vi "Desplegar arreglos boleanos.vi"(8 "error in (no error)":errorcluster, 10 "Expected Response out":string, 11 "Simulado in":refnum<class "Simulado.lvclass">) -> (0 "error out":errorcluster, 1 "Puerto":string, 2 "output array":bool[](array[boolean]), 3 "Simulado out":refnum<class "Simulado.lvclass">)   [LabVIEW 2020, in "Simulado.lvclass"]
uses:
  Simulado.lvclass
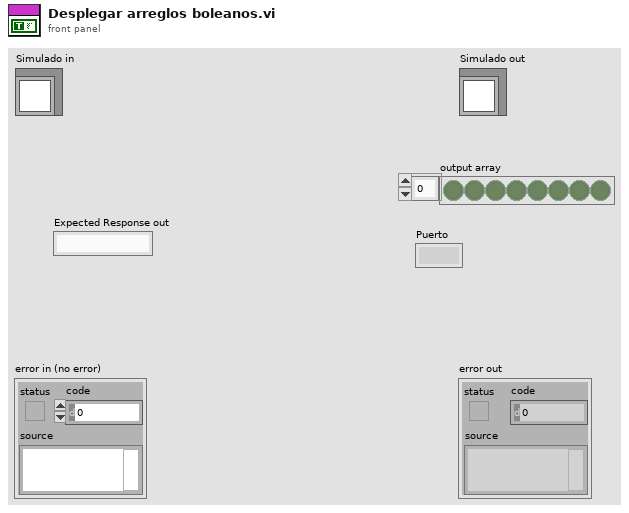
[diagram p1: front panel]
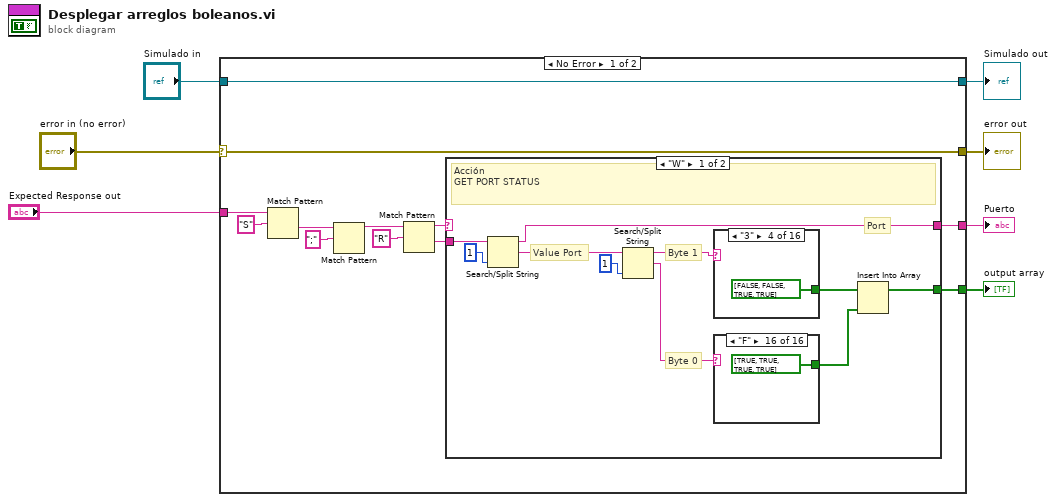
[diagram p0: block diagram]
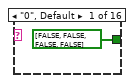
[diagram p2: hidden frame]
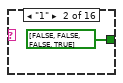
[diagram p3: hidden frame]
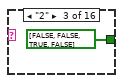
[diagram p4: hidden frame]
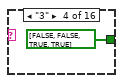
[diagram p5: hidden frame]
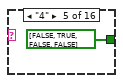
[diagram p6: hidden frame]
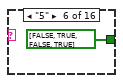
[diagram p7: hidden frame]
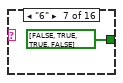
[diagram p8: hidden frame]
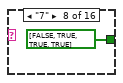
[diagram p9: hidden frame]
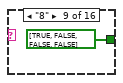
[diagram p10: hidden frame]
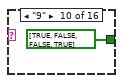
[diagram p11: hidden frame]
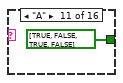
[diagram p12: hidden frame]
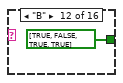
[diagram p13: hidden frame]
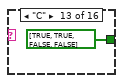
[diagram p14: hidden frame]
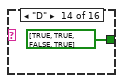
[diagram p15: hidden frame]
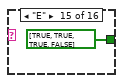
[diagram p16: hidden frame]
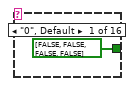
[diagram p17: hidden frame]
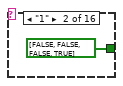
[diagram p18: hidden frame]
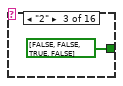
[diagram p19: hidden frame]
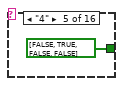
[diagram p20: hidden frame]
diagram:
  n1 = case shown="No Error" "error in (no error)" {
    selector: "error in (no error)" -> [w18 w65]
    tunnel: [w18 w65] -> w4
    tunnel: [w19 w64] -> w3
    tunnel: "Simulado in" -> [w19 w64]
    tunnel: [w10 _] -> w1
    tunnel: [w9 _] -> w2
    tunnel: "Expected Response out" -> [w8 _]
    frame No Error {
      n2 = Match Pattern(string=w8, regular expression="S") -> (after substring=w15:string)  [unwired: 1 in, 3 out]
      n3 = Match Pattern(string=w15, regular expression=";") -> (before substring=w14:string)  [unwired: 1 in, 3 out]
      n4 = Match Pattern(string=w14, regular expression="R" ("search string/char (-)")) -> (before substring=w12:string, after substring=w11:string)  [unwired: 1 in, 2 out]
      n5 = case shown="\"W\"" w12 {
        tunnel: w11 -> [w29 _]
        tunnel: [w27 "" ("Expected Response out")] -> w10
        tunnel: [w20 bool[] [FALSE, FALSE, FALSE, FALSE, FALSE, FALSE, FALSE, FALSE]] -> w9
        frame "W" {
          # "Byte 0"
          # "Byte 1"
          # "Value Port"
          # "Port"
          # "Acción\nGET PORT STATUS"
          n6 = Search/Split String(string=w29, offset (0)=1) -> (substring before match=w27:string, match + rest of string=w26:string)  [unwired: 1 in, 1 out]
          n7 = Search/Split String(string=w26, offset (0)=1) -> (substring before match=w24:string, match + rest of string=w23:string)  [unwired: 1 in, 1 out]
          n8 = case shown="\"3\"" w24 {
            tunnel: [bool[] [FALSE, FALSE, FALSE, FALSE] bool[] [FALSE, FALSE, FALSE, TRUE] bool[] [FALSE, FALSE, TRUE, FALSE] bool[] [FALSE, FALSE, TRUE, TRUE] bool[] [FALSE, TRUE, FALSE, FALSE] bool[] [FALSE, TRUE, FALSE, TRUE] bool[] [FALSE, TRUE, TRUE, FALSE] bool[] [FALSE, TRUE, TRUE, TRUE] bool[] [TRUE, FALSE, FALSE, FALSE] bool[] [TRUE, FALSE, FALSE, TRUE] bool[] [TRUE, FALSE, TRUE, FALSE] bool[] [TRUE, FALSE, TRUE, TRUE] bool[] [TRUE, TRUE, FALSE, FALSE] bool[] [TRUE, TRUE, FALSE, TRUE] bool[] [TRUE, TRUE, TRUE, FALSE] bool[] [TRUE, TRUE, TRUE, TRUE]] -> w22
            frame "0", Default {
            }
            frame "1" {
            }
            frame "2" {
            }
            frame "3" {
            }
            frame "4" {
            }
            frame "5" {
            }
            frame "6" {
            }
            frame "7" {
            }
            frame "8" {
            }
            frame "9" {
            }
            frame "A" {
            }
            frame "B" {
            }
            frame "C" {
            }
            frame "D" {
            }
            frame "E" {
            }
            frame "F" {
            }
          }
          n9 = case shown="\"F\"" w23 {
            tunnel: [bool[] [FALSE, FALSE, FALSE, FALSE] bool[] [FALSE, FALSE, FALSE, TRUE] bool[] [FALSE, FALSE, TRUE, FALSE] bool[] [FALSE, FALSE, TRUE, TRUE] bool[] [FALSE, TRUE, FALSE, FALSE] bool[] [FALSE, TRUE, FALSE, TRUE] bool[] [FALSE, TRUE, TRUE, FALSE] bool[] [FALSE, TRUE, TRUE, TRUE] bool[] [TRUE, FALSE, FALSE, FALSE] bool[] [TRUE, FALSE, FALSE, TRUE] bool[] [TRUE, FALSE, TRUE, FALSE] bool[] [TRUE, FALSE, TRUE, TRUE] bool[] [TRUE, TRUE, FALSE, FALSE] bool[] [TRUE, TRUE, FALSE, TRUE] bool[] [TRUE, TRUE, TRUE, FALSE] bool[] [TRUE, TRUE, TRUE, TRUE]] -> w21
            frame "0", Default {
            }
            frame "1" {
            }
            frame "2" {
            }
            frame "3" {
            }
            frame "4" {
            }
            frame "5" {
            }
            frame "6" {
            }
            frame "7" {
            }
            frame "8" {
            }
            frame "9" {
            }
            frame "A" {
            }
            frame "B" {
            }
            frame "C" {
            }
            frame "D" {
            }
            frame "E" {
            }
            frame "F" {
            }
          }
          n10 = Insert Into Array(array=w22, new element=w21) -> (w20:bool[])  [unwired: 1 in]
        }
        frame Default {
          # "Cualquier otro"
        }
      }
    }
    frame Error {
    }
  }
  "error out" <- w4
  "Simulado out" <- w3
  "Puerto" <- w1
  "output array" <- w2
